vi "WriteRead.vi"(5 "Add <n>?":bool, 6 "Bytes to Read":u32, 7 "Command to Send":string, 8 "Error In":errorcluster, 9 "Send Command":bool, 10 "UART Channel (0)":u8, 11 "LINX Resource":T1) -> (0 "Error Out":errorcluster, 2 "Data":string, 3 "LINX Resource":T1)   [LabVIEW 2014, in "LMH-LINX.lvlib" / "PmodBT2.lvlib"]
doc: "Optionally send a command to the PmodBT2, then read the specified number of bytes from the PmodBT2."
uses:
  <vilib>/MakerHub/LINX/Public/Sensors/Pmods/BT2/PmodBT2.lvlib
  <vilib>/MakerHub/LINX/Private/Type Defs/LINX Ref.ctl
  <vilib>/MakerHub/LINX/Private/Type Defs/Platform.ctl
  <vilib>/MakerHub/LINX/Private/Type Defs/Interface.ctl
  <vilib>/MakerHub/LINX/Private/Device/Type Defs/LINX Device Config.ctl
  <vilib>/MakerHub/LINX/Private/Device/Type Defs/TCP Config.ctl
  <vilib>/MakerHub/LINX/Private/Device/Type Defs/Channels.ctl
  <vilib>/MakerHub/LINX/Public/Peripherals/UART/UART Write Byte Array.vi
  <vilib>/MakerHub/LINX/Private/Local IO/LinxUartWrite.vi
  <vilib>/MakerHub/LINX/Public/Utilities/Check Channel.vi
  <vilib>/MakerHub/LINX/Private/Utilties/Generate Error.vi
  <vilib>/MakerHub/LINX/Public/Peripherals/UART/UART Read String.vi
  <vilib>/MakerHub/LINX/LMH-LINX.lvlib
  <vilib>/MakerHub/LINX/Private/Device/Device.lvlib
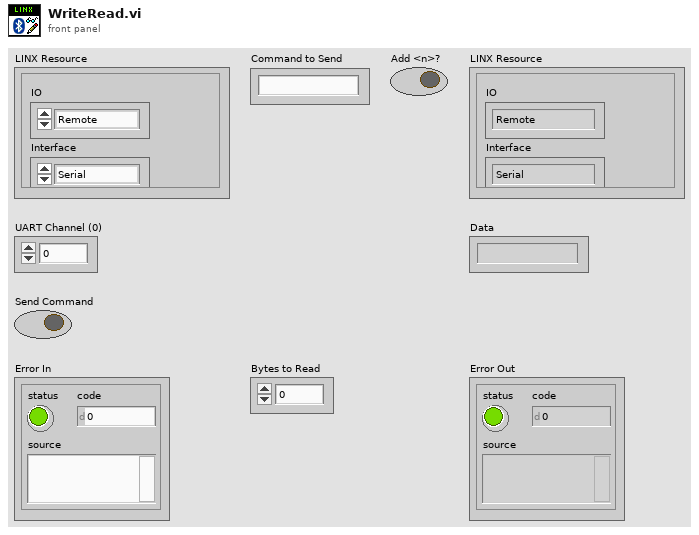
[diagram p1: front panel]
types:
  T1 = typedef "LMH-LINX.lvlib/LINX Ref.ctl" = cluster{"IO":T2, "Interface":T3, "LINX Device Config":T4}
  T2 = typedef "LMH-LINX.lvlib/Platform.ctl" = enum16{"Remote", "Local"}
  T3 = typedef "LMH-LINX.lvlib/Interface.ctl" = enum16{"Serial", "TCP"}
  T4 = typedef "LMH-LINX.lvlib/Device.lvlib/LINX Device Config.ctl" = cluster{"Interface":T3, "COM Port":refnum<visa-resource-name>, "TCP Configuration":T5, "Device Family":u8, "Device ID":u8, "Device Name":string, "TCP Ref":refnum<k5>, "Channels":T6}
  T5 = typedef "LMH-LINX.lvlib/Device.lvlib/TCP Config.ctl" = cluster{"IP Address":string, "Port":u16}
  T6 = typedef "LMH-LINX.lvlib/Channels.ctl" = cluster{"DI":u8[], "DO":u8[], "AI":u8[], "AO":u8[], "PWM":u8[], "QE":u8[], "UART":u8[], "I2C 2":u8[], "SPI":u8[], "CAN":u8[], "Servo":u8[], "AI Ref (V)":dbl, "AI Resolution (Bits)":u8, "AO Ref (V)":dbl, "AO Resolution (Bits)":u8}
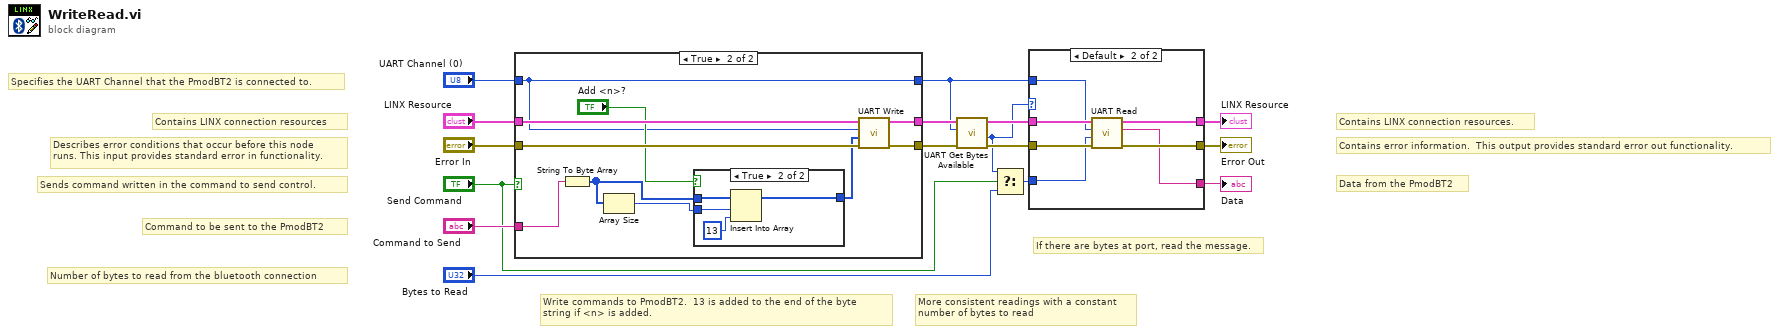
[diagram p0: block diagram]
diagram:
  # "Data from the PmodBT2"
  # "Contains error information.  This output provides standard error out functionality."
  # "Contains LINX connection resources."
  # "Number of bytes to read from the bluetooth connection"
  # "Command to be sent to the PmodBT2"
  # "Sends command written in the command to send control."
  # "Describes error conditions that occur before this node\nruns. This input provides standard error in functionality."
  # "Contains LINX connection resources"
  # "Specifies the UART Channel that the PmodBT2 is connected to."
  # "If there are bytes at port, read the message."
  # "More consistent readings with a constant\nnumber of bytes to read"
  # "Write commands to PmodBT2.  13 is added to the end of the byte \nstring if <n> is added."
  n1 = case shown="True" "Send Command" {
    tunnel: "Error In" -> [w18 w29]
    tunnel: [w18 w28] -> w9
    tunnel: [w19 w27] -> w10
    tunnel: "LINX Resource" -> [w19 w26]
    tunnel: "UART Channel (0)" -> [w17 w20]
    tunnel: "Command to Send" -> [_ w21]
    tunnel: [w17 w20] -> w8
    frame False {
    }
    frame True {
      n2 = String To Byte Array(string=w21) -> (unsigned byte array=w24:u8[])
      n3 = Array Size(array=w24) -> (size(s)=w23:i32)
      n4 = case shown="True" "Add <n>?" {
        tunnel: w24 -> [w30 w34]
        tunnel: w23 -> [_ w33]
        tunnel: [w30 w31] -> w22
        frame False {
        }
        frame True {
          n5 = Insert Into Array(array=w34, index=w33, new element=u8 13 ("new element/subarray")) -> (w31:u8[])
        }
      }
      n6 = call-poly <vilib>:"UART Write.vi"("Error In"=w29, "Data"=w22, "UART Channel (0)"=w20, "LINX Resource"=w26) -> ("Error Out"=w28:errorcluster, "LINX Resource"=w27:T1)  [unwired: 6 in]
    }
  }
  n7 = call <vilib>:"UART Get Bytes Available.vi"("Error In"=w9, "UART Channel (0)"=w8, "LINX Resource"=w10) -> ("Error Out"=w11:errorcluster, "Bytes Available"=w2:u8, "LINX Resource"=w12:T1)  [unwired: 6 in]
  n8 = Select(t=w2, s="Send Command", f="Bytes to Read") -> (s? t:f=w4:u32)
  n9 = case shown="Default" w2 {
    tunnel: w12 -> [w36 w43]
    tunnel: w11 -> [w35 w42]
    tunnel: [w36 w41] -> w7
    tunnel: [w35 w40] -> w6
    tunnel: w8 -> [_ w39]
    tunnel: w4 -> [_ w38]
    tunnel: [_ w37] -> w1
    frame 0 {
    }
    frame Default {
      n10 = call-poly <vilib>:"UART Read.vi"("Error In"=w42, "Num Bytes"=w38, "UART Channel (0)"=w39, "LINX Resource"=w43) -> ("Error Out"=w40:errorcluster, "Data"=w37:string, "LINX Resource"=w41:T1)  [unwired: 5 in]
    }
  }
  "LINX Resource" <- w7
  "Error Out" <- w6
  "Data" <- w1
